vi "liblinear_crossvalidation_example.vi"(8 "error in (no error)":errorcluster) -> (0 "error out":errorcluster, 3 "Binary Confusion Matrix":T1)   [LabVIEW 2015]
uses:
  Tools/Controls/Binary_ConfusionMatrix.ctl
  Controls/liblinear_problem.ctl
  LibSVM Sparse/Wrapper API/Controls/svm_node.ctl
  Controls/liblinear_parameter.ctl
  Controls/liblinear_solver.ctl
  Tools/SubVIs/Sparse - Scale Problem Linear.vi
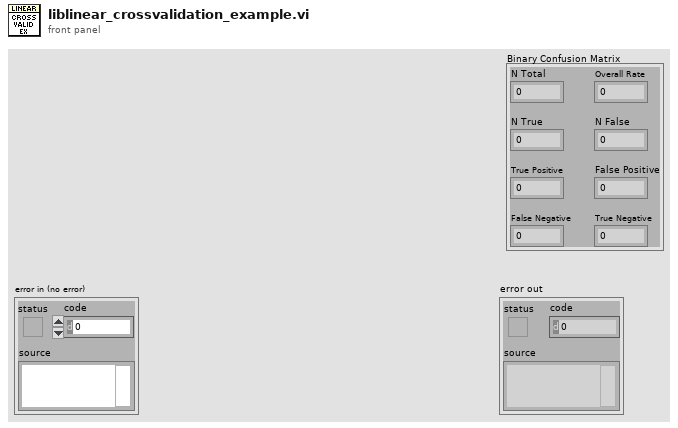
[diagram p1: front panel]
types:
  T1 = typedef "Binary_ConfusionMatrix.ctl" = cluster{"N Total":u32, "N True":u32, "N False":u32, "Overall Rate":dbl, "True Positive":dbl, "False Positive":dbl, "False Negative":dbl, "True Negative":dbl}
  T2 = typedef "liblinear_parameter.ctl" = cluster{"solver_type":T3, "eps":dbl, "C":dbl, "weight_label":i32[], "weight":dbl[], "p":dbl}
  T3 = typedef "liblinear_solver.ctl" = u32
  T4 = typedef "liblinear_problem.ctl" = cluster{"y":dbl[], "x":cluster{T5[]}[], "bias":dbl}
  T5 = typedef "svm_node.ctl" = cluster{"index":i32, "value":dbl}
  T6 = typedef "svm_problem.ctl" = cluster{"y":dbl[], "x":cluster{T5[]}[]}
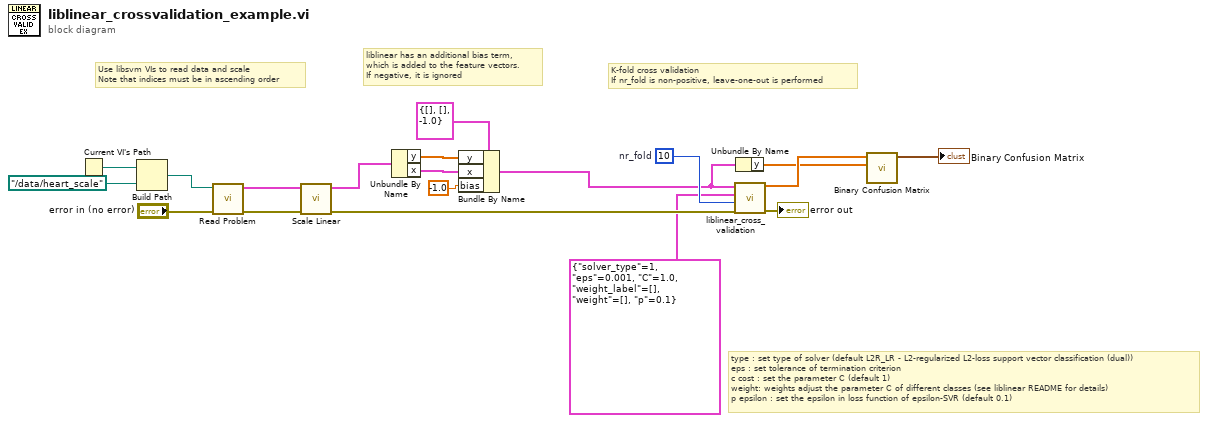
[diagram p0: block diagram]
diagram:
  w15 = 10  # nr_fold
  # "K-fold cross validation\nIf nr_fold is non-positive, leave-one-out is performed"
  # "type : set type of solver (default L2R_LR - L2-regularized L2-loss support vector classification (dual))\neps : set tolerance of termination criterion\nc cost : set the parameter C (default 1)\nweight: weights adjust the parameter C of different classes (see liblinear README for details)\np epsilon : set the epsilon in loss function of epsilon-SVR (default 0.1)"
  # "liblinear has an additional bias term, \nwhich is added to the feature vectors.\nIf negative, it is ignored"
  # "Use libsvm VIs to read data and scale\nNote that indices must be in ascending order"
  n1 = Current VI's Path() -> (path=w19:path)
  n2 = Build Path(base path=w19, name or relative path=path "../data/heart_scale" ("file path (use dialog)")) -> (appended path=w17:path)
  n3 = call "Read Problem.vi"("error in (no error)"="error in (no error)", "file path (use dialog)"=w17) -> ("error out"=w16:errorcluster, "svm_problem"=w2:T6)  [unwired: 8 in]
  n4 = call-poly "Scale Linear.vi"("error in (no error)"=w16, "Problem"=w2) -> ("error out"=w10:errorcluster, "Scaled problem"=w1:T6)  [unwired: 7 in, 1 out]
  n5 = Unbundle By Name(w1) -> ("y"=w13:dbl[], "x"=w12:cluster{T5[]}[])
  n6 = Bundle By Name(cluster=T4 {"y"=[], "x"=[], "bias"=-1.0} ("liblinear_problem"), "y"=w13, "x"=w12, "bias"=-1.0) -> (w4:T4)
  n7 = call "liblinear_cross_validation.vi"("error in (no error)"=w10, "nr_fold"=w15, "parameters"=T2 {"solver_type"=1, "eps"=0.001, "C"=1.0, "weight_label"=[], "weight"=[], "p"=0.1}, "problem"=w4) -> ("error out"=→"error out":errorcluster, "target"=w8:dbl[])  [unwired: 6 in]
  n8 = Unbundle By Name(w4) -> ("y"=w7:dbl[])
  n9 = call "Binary Confusion Matrix.vi"("Actual Labels"=w7, "Predicted Labels"=w8) -> ("Binary Confusion Matrix"=→"Binary Confusion Matrix":T1)  [unwired: 8 in, 1 out]
